vi "Channels.vi"(1 "Input":string, 2 "Channel FGV Selector":T2, 3 "Action":T1) -> (0 "Output":string)   [LabVIEW 2013]
uses:
  Channel FGV Selector.ctl
  Action.ctl
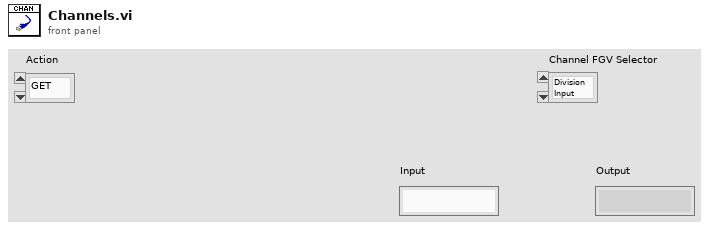
[diagram p1: front panel]
types:
  T1 = typedef "Action.ctl" = enum16{"GET", "PUT", "DELETE"}
  T2 = typedef "Channel FGV Selector.ctl" = enum16{"Division Input", "Sum Input", "Z Output", "Z Input", "Y Output", "Y Input", "X Output", "X Input"}
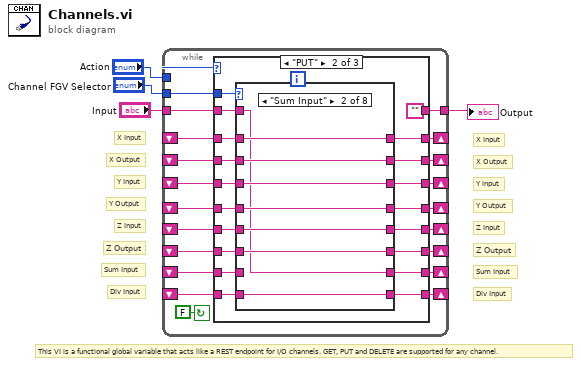
[diagram p0: block diagram]
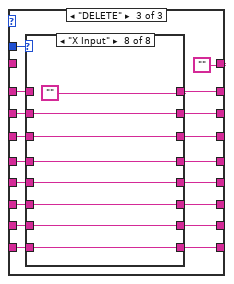
[diagram p17: hidden frame]
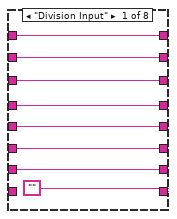
[diagram p18: hidden frame]
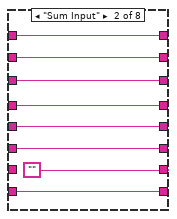
[diagram p19: hidden frame]
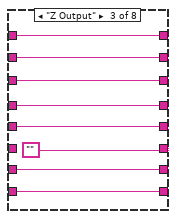
[diagram p20: hidden frame]
diagram:
  # "This VI is a functional global variable that acts like a REST endpoint for I/O channels. GET, PUT and DELETE are supported for any channel."
  # "Div Input"
  # "Sum Input"
  # "Z Output"
  # "Y Output"
  # "X Output"
  # "Z Input"
  # "Y Input"
  # "X Input"
  # "Div Input"
  # "Sum Input"
  # "Z Output"
  # "Y Output"
  # "X Output"
  # "Z Input"
  # "Y Input"
  # "X Input"
  n1 = while {
    shift-right: [w23] -> _
    shift-left: _ -> [w24]
    shift-right: [w22] -> _
    shift-left: _ -> [w21]
    shift-right: [w20] -> _
    shift-left: _ -> [w19]
    shift-right: [w18] -> _
    shift-left: _ -> [w17]
    shift-right: [w16] -> _
    shift-left: _ -> [w15]
    shift-right: [w14] -> _
    shift-left: _ -> [w13]
    shift-right: [w12] -> _
    shift-left: _ -> [w11]
    shift-right: [w10] -> _
    shift-left: _ -> [w9]
    tunnel: "Input" -> [w7]
    tunnel: [w8] -> w3
    tunnel: "Channel FGV Selector" -> [w6]
    tunnel: "Action" -> [w5]
    stop <- FALSE continue-if-true
    n2 = case shown="\"PUT\"" w5 {
      tunnel: w6 -> [w43 w126 w208]
      tunnel: w24 -> [w35 w123 w207]
      tunnel: [w27 w124 w206] -> w23
      tunnel: [w28 w122 w205] -> w22
      tunnel: w21 -> [w36 w121 w204]
      tunnel: [w29 w120 w203] -> w20
      tunnel: w19 -> [w37 w119 w202]
      tunnel: [w30 w118 w201] -> w18
      tunnel: w17 -> [w38 w117 w200]
      tunnel: [w31 w116 w199] -> w16
      tunnel: w15 -> [w39 w115 w198]
      tunnel: [w32 w114 w197] -> w14
      tunnel: w13 -> [w40 w113 w196]
      tunnel: [w33 w112 w195] -> w12
      tunnel: w11 -> [w42 w111 w194]
      tunnel: [w34 w109 w193] -> w10
      tunnel: w9 -> [w41 w110 w192]
      tunnel: [w26 "" ""] -> w8
      tunnel: w7 -> [_ w108 _]
      frame "GET", Default {
        n3 = case shown="\"Division Input\"" w43 {
          tunnel: w42 -> [w45 w52 w62 w70 w78 w86 w94 w102]
          tunnel: w41 -> [w44 w59 w61 w69 w77 w85 w93 w101]
          tunnel: w40 -> [w46 w58 w60 w71 w79 w87 w95 w103]
          tunnel: w39 -> [w47 w57 w63 w68 w80 w88 w96 w104]
          tunnel: w38 -> [w48 w56 w64 w72 w76 w89 w97 w105]
          tunnel: w37 -> [w49 w55 w65 w73 w81 w84 w98 w106]
          tunnel: w36 -> [w50 w54 w66 w74 w82 w90 w92 w107]
          tunnel: w35 -> [w51 w53 w67 w75 w83 w91 w99 w100]
          tunnel: [w44 w59 w61 w69 w77 w85 w93 w101] -> w34
          tunnel: [w45 w52 w62 w70 w78 w86 w94 w102] -> w33
          tunnel: [w46 w58 w60 w71 w79 w87 w95 w103] -> w32
          tunnel: [w47 w57 w63 w68 w80 w88 w96 w104] -> w31
          tunnel: [w48 w56 w64 w72 w76 w89 w97 w105] -> w30
          tunnel: [w49 w55 w65 w73 w81 w84 w98 w106] -> w29
          tunnel: [w50 w54 w66 w74 w82 w90 w92 w107] -> w28
          tunnel: [w51 w53 w67 w75 w83 w91 w99 w100] -> w27
          tunnel: [w44 w52 w60 w68 w76 w84 w92 w100] -> w26
          frame "Division Input" {
          }
          frame "Sum Input" {
          }
          frame "Z Output" {
          }
          frame "Z Input" {
          }
          frame "Y Output" {
          }
          frame "Y Input" {
          }
          frame "X Output" {
          }
          frame "X Input" {
          }
        }
      }
      frame "PUT" {
        n4 = case shown="\"Sum Input\"" w126 {
          tunnel: [w134 w142 w143 w154 w163 w173 w181 w190] -> w124
          tunnel: w123 -> [w134 w142 w143 w154 w163 w173 w181 _]
          tunnel: [w133 w141 w144 w155 w164 w172 w182 w189] -> w122
          tunnel: w121 -> [w133 w141 w144 w155 w164 w172 _ w189]
          tunnel: [w132 w140 w145 w156 w165 w174 w180 w188] -> w120
          tunnel: w119 -> [w132 w140 w145 w156 w165 _ w180 w188]
          tunnel: [w131 w139 w146 w157 w166 w171 w179 w187] -> w118
          tunnel: w117 -> [w131 w139 w146 w157 _ w171 w179 w187]
          tunnel: [w130 w138 w147 w158 w162 w170 w178 w186] -> w116
          tunnel: w115 -> [w130 w138 w147 _ w162 w170 w178 w186]
          tunnel: [w129 w137 w148 w153 w161 w169 w177 w185] -> w114
          tunnel: w113 -> [w129 w137 _ w153 w161 w169 w177 w185]
          tunnel: [w128 w136 w149 w152 w160 w168 w176 w184] -> w112
          tunnel: w111 -> [w128 _ w149 w152 w160 w168 w176 w184]
          tunnel: w110 -> [_ w135 w150 w151 w159 w167 w175 w183]
          tunnel: [w127 w135 w150 w151 w159 w167 w175 w183] -> w109
          tunnel: w108 -> [w127 w136 w148 w158 w166 w174 w182 w190]
          frame "Division Input" {
          }
          frame "Sum Input" {
          }
          frame "Z Output" {
          }
          frame "Z Input" {
          }
          frame "Y Output" {
          }
          frame "Y Input" {
          }
          frame "X Output" {
          }
          frame "X Input" {
          }
        }
      }
      frame "DELETE" {
        n5 = case shown="\"X Input\"" w208 {
          tunnel: w207 -> [w216 w218 w225 w236 w245 w254 w263 _]
          tunnel: [w216 w218 w225 w236 w245 w254 w263 ""] -> w206
          tunnel: [w215 w219 w226 w237 w246 w255 "" w271] -> w205
          tunnel: w204 -> [w215 w219 w226 w237 w246 w255 _ w271]
          tunnel: [w214 w220 w227 w238 w247 "" w262 w270] -> w203
          tunnel: w202 -> [w214 w220 w227 w238 w247 _ w262 w270]
          tunnel: [w213 w221 w228 w239 "" w253 w261 w269] -> w201
          tunnel: w200 -> [w213 w221 w228 w239 _ w253 w261 w269]
          tunnel: [w212 w222 w231 "" w244 w252 w260 w268] -> w199
          tunnel: w198 -> [w212 w222 w231 _ w244 w252 w260 w268]
          tunnel: [w211 w223 "" w235 w243 w251 w259 w267] -> w197
          tunnel: w196 -> [w211 w223 _ w235 w243 w251 w259 w267]
          tunnel: [w210 "" w230 w234 w242 w250 w258 w266] -> w195
          tunnel: w194 -> [w210 _ w230 w234 w242 w250 w258 w266]
          tunnel: ["" w217 w229 w233 w241 w249 w257 w265] -> w193
          tunnel: w192 -> [_ w217 w229 w233 w241 w249 w257 w265]
          frame "Division Input" {
          }
          frame "Sum Input" {
          }
          frame "Z Output" {
          }
          frame "Z Input" {
          }
          frame "Y Output" {
          }
          frame "Y Input" {
          }
          frame "X Output" {
          }
          frame "X Input" {
          }
        }
      }
    }
  }
  "Output" <- w3
